vi "ConfigureAquisition.vi"(8 "Acquisition":T1={"Sample Rate"=100000000.0, "Clock mode"=enum."Internal", "Mode"=0, "Depth"=8192.0, "Segment Size"=8192.0, "Trigger Timeout"=1000000.0, "Trigger Holdoff"=0.0, "Trigger Delay"=0.0} {"Segment Size" min=256.0 step=128.0; "Trigger Holdoff" min=0.0 step=128.0; "Trigger Delay" min=0.0 step=128.0; "Depth" min=256.0 step=128.0; "Mode" items=["Single", "Dual", "Quad", "Octal"]}, 9 "Trigger":T4={"Slope"=0, "Level"=0, "Source"=0, "External Range"=2000, "External Coupling"=0, "External"=FALSE, "Disable"=FALSE, "External Impedance"=1} {"External Impedance" items=["50 Ohm", "HiZ"]; "External Coupling" items=["DC", "AC"]; "External Range" min=2000 max=10000 step=8000; "Slope" items=["Rising", "Falling"]; "Level" min=-100 max=100; "Source" min=0 max=64 step=1}, 10 "channels configuration":T3(array[cluster])=[{"Coupling"=0, "Differential Input"=FALSE, "Direct-to-ADC"=FALSE, "Range"=2000, "Impedance"=50, "DC Offset"=0}, {"Coupling"=0, "Differential Input"=FALSE, "Direct-to-ADC"=FALSE, "Range"=2000, "Impedance"=50, "DC Offset"=0}, {"Coupling"=0, "Differential Input"=FALSE, "Direct-to-ADC"=FALSE, "Range"=2000, "Impedance"=50, "DC Offset"=0}, {"Coupling"=0, "Differential Input"=FALSE, "Direct-to-ADC"=FALSE, "Range"=2000, "Impedance"=50, "DC Offset"=0}] {"Impedance" min=50 max=1000000 step=999950; "Coupling" items=["DC", "AC"]}, 11 "Handle Cluster":T2) -> (0 "Error Code":i32, 3 "Handle Cluster 2":T2)   [LabVIEW 2015]
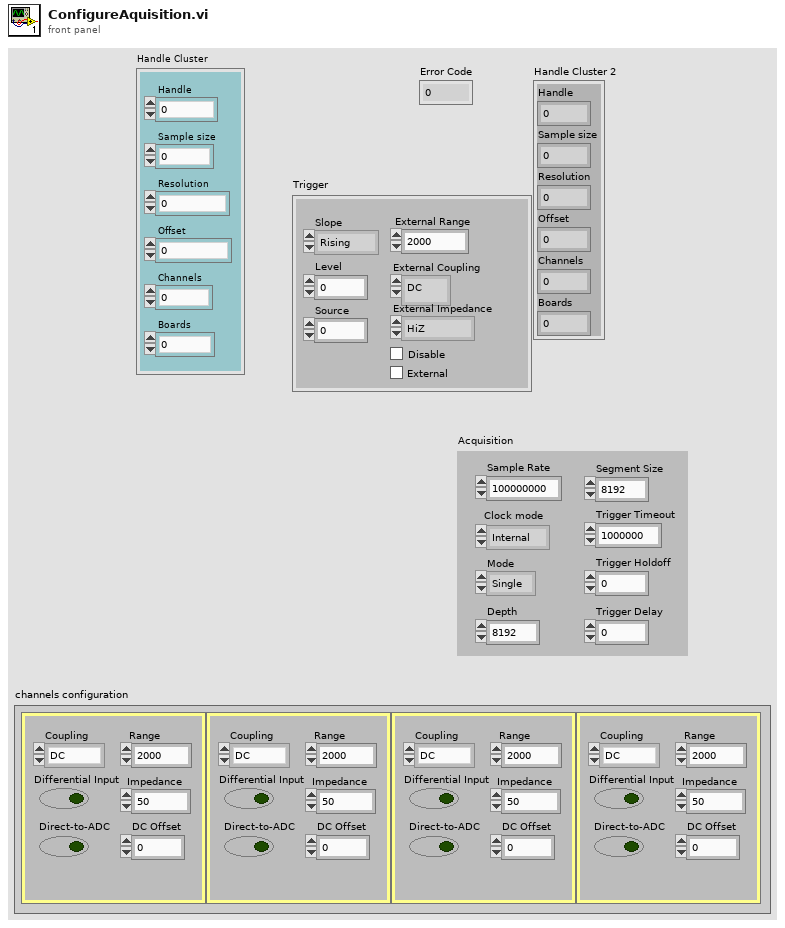
[diagram p1: front panel]
types:
  T1 = cluster{"Sample Rate":dbl, "Clock mode":enum16{"Internal", "External", "Reference"}, "Mode":u16, "Depth":dbl, "Segment Size":dbl, "Trigger Timeout":dbl, "Trigger Holdoff":dbl, "Trigger Delay":dbl}
  T2 = cluster{"Handle":u32, "Sample size":u32, "Resolution":i32, "Offset":i32, "Channels":u32, "Boards":u32}
  T3 = cluster{"Coupling":u16, "Differential Input":bool, "Direct-to-ADC":bool, "Range":u32, "Impedance":u32, "DC Offset":i32}[]
  T4 = cluster{"Slope":u16, "Level":i32, "Source":i32, "External Range":u32, "External Coupling":u16, "External":bool, "Disable":bool, "External Impedance":u16}
  T5 = cluster{string, "Differential Input":bool, "Direct-to-ADC":bool, "Range":u32, "Impedance":u32, "DC Offset":i32, u32}
  T6 = cluster{"RingText.Text":string, "Level":i32, "Source":i32, "External Range":u32, "RingText.Text":string, "External":bool, "Disable":bool, "RingText.Text":string}
  T7 = cluster{"RingText.Text":string, "Level":i32, "Source":i32, "External Range":u32, "RingText.Text":string, "External":bool, "Disable":bool, "RingText.Text":string}[]
  T8 = cluster{"Sample Rate":dbl, "Clock mode":enum16{"Internal", "External", "Reference"}, "RingText.Text":string, "Depth":dbl, "Segment Size":dbl, "Trigger Timeout":dbl, "Trigger Holdoff":dbl, "Trigger Delay":dbl}
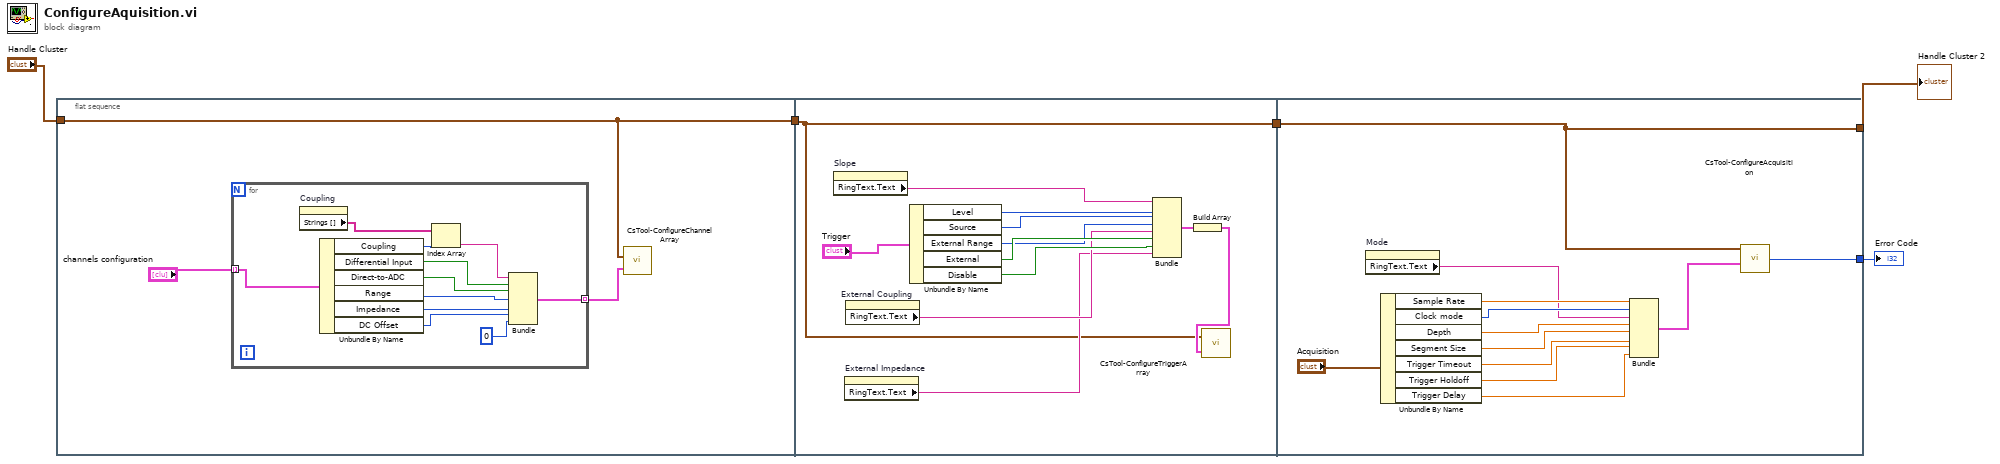
[diagram p0: block diagram]
diagram:
  n1 = flat-sequence {
    tunnel: "Handle Cluster" -> [w6]
    tunnel: [w6] -> w4
    tunnel: w4 -> [w20]
    tunnel: [w20] -> w3
    tunnel: w3 -> [w43]
    tunnel: [w43] -> w2
    tunnel: [w32] -> w1
    frame #0 {
      n2 = for {
        tunnel: "channels configuration" -> [w11] mode=indexing
        tunnel: [w9] -> w7 mode=indexing
        n3 = property on="Coupling" class="Ring (strict)"() -> ("Strings []"=w10:string[])  [unwired: 2 in, 2 out]
        n4 = Unbundle By Name(w11) -> ("Coupling"=w15:u16, "Differential Input"=w12:bool, "Direct-to-ADC"=w16:bool, "Range"=w17:u32, "Impedance"=w18:u32, "DC Offset"=w19:i32)
        n5 = Index Array(array=w10, index=w15) -> (element=w13:string)
        n6 = Bundle(w13, "Differential Input"=w12, "Direct-to-ADC"=w16, "Range"=w17, "Impedance"=w18, "DC Offset"=w19, u32 0) -> (w9:T5)  [unwired: 1 in]
      }
      n7 = call <userlib>:"CsTool-ConfigureChannelArray.vi"("Channels"=w7, "Handle Cluster"=w6) -> ()  [unwired: 1 out]
    }
    frame #1 {
      n8 = property on="Slope" class="Ring (strict)"() -> ("RingText.Text"=w25:string)  [unwired: 2 in, 2 out]
      n9 = property on="External Impedance" class="Ring (strict)"() -> ("RingText.Text"=w23:string)  [unwired: 2 in, 2 out]
      n10 = property on="External Coupling" class="Ring (strict)"() -> ("RingText.Text"=w29:string)  [unwired: 2 in, 2 out]
      n11 = Unbundle By Name("Trigger") -> ("Level"=w26:i32, "Source"=w27:i32, "External Range"=w28:u32, "External"=w30:bool, "Disable"=w31:bool)
      n12 = Bundle("RingText.Text"=w25, "Level"=w26, "Source"=w27, "External Range"=w28, "RingText.Text"=w29, "External"=w30, "Disable"=w31, "RingText.Text"=w23) -> (w22:T6)  [unwired: 1 in]
      n13 = Build Array(w22) -> (w21:T7)
      n14 = call <userlib>:"CsTool-ConfigureTriggerArray.vi"("Triggers"=w21, "Handle Cluster"=w20) -> ()  [unwired: 1 out]
    }
    frame #2 {
      n15 = property on="Mode" class="Ring (strict)"() -> ("RingText.Text"=w34:string)  [unwired: 2 in, 2 out]
      n16 = Unbundle By Name("Acquisition") -> ("Sample Rate"=w36:dbl, "Clock mode"=w37:enum16{"Internal", "External", "Reference"}, "Depth"=w42:dbl, "Segment Size"=w40:dbl, "Trigger Timeout"=w41:dbl, "Trigger Holdoff"=w39:dbl, "Trigger Delay"=w35:dbl)
      n17 = Bundle("Sample Rate"=w36, "Clock mode"=w37, "RingText.Text"=w34, "Depth"=w42, "Segment Size"=w40, "Trigger Timeout"=w41, "Trigger Holdoff"=w39, "Trigger Delay"=w35) -> (w33:T8)  [unwired: 1 in]
      n18 = call <userlib>:"CsTool-ConfigureAcquisition.vi"("Handle Cluster"=w43, "Acquisition"=w33) -> ("Error Code"=w32:i32)  [unwired: 3 in]
    }
  }
  "Handle Cluster 2" <- w2
  "Error Code" <- w1
